vi "Get Controls RegisterMap.vi"(8 "error in (no error)":errorcluster, 11 "Item Ref in":T3 format="%.0x") -> (0 "error out":errorcluster, 2 "Controls RegisterMap":T1[](array[typedef]) {"fgpa cd ref" format="%.0x"; "reserver ref" format="%.0x"}, 3 "Item Ref out":T3 format="%.0x")   [LabVIEW 2016]
uses:
  <vilib>/NI VeriStand/Custom Device API/Custom Device API.lvlib
  <vilib>/NI Veristand/Custom Device API/Get Item Property (Variant).vi
  SubVIs/Channel Type.ctl
  FPGA Addon System Explorer.lvlib
  <vilib>/NI Veristand/Custom Device API/Custom Device Item Ref.ctl
  SubVIs/fpga resource.ctl
  VeriStand-FPGA-Resource-Manager/Source/FPGA Resource Manager System Definition.lvlib
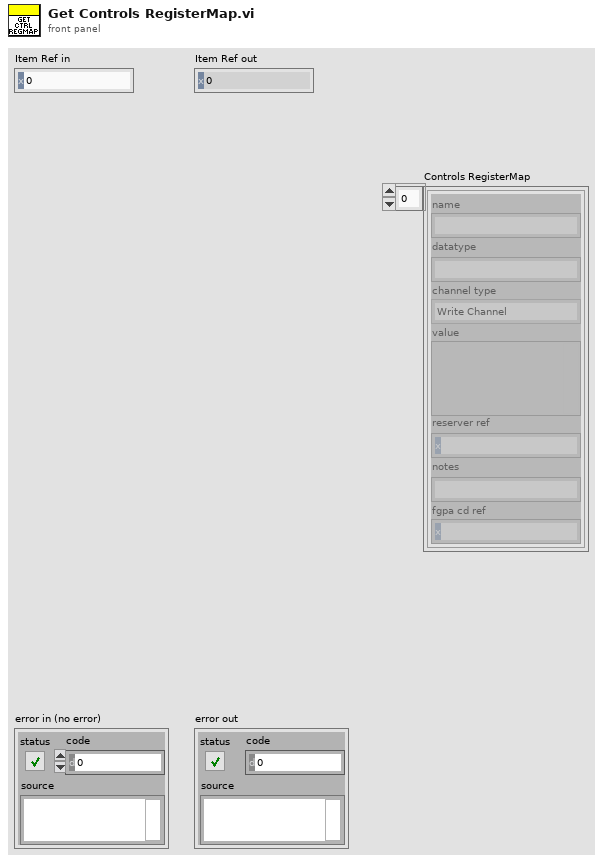
[diagram p1: front panel]
types:
  T1 = typedef "FPGA Addon System Explorer.lvlib/fpga resource.ctl" = cluster{"name":string, "datatype":string, "channel type":T2, "value":variant, "reserver ref":T3, "notes":string, "fgpa cd ref":T3}
  T2 = typedef "FPGA Addon System Explorer.lvlib/Channel Type.ctl" = enum16{"Write Channel", "Read Channel", "Write Waveform", "Read Waveform"}
  T3 = typedef "Custom Device API.lvlib/Custom Device Item Ref.ctl" = u64
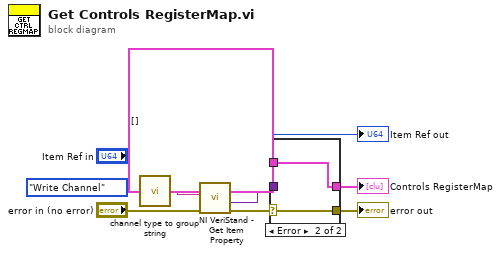
[diagram p0: block diagram]
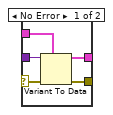
[diagram p2: hidden frame]
diagram:
  n1 = call "channel type to group string.vi"("channel type"=Channel_Type."Write Channel") -> ("FPGA.Controls"=w3:string)  [unwired: 10 in]
  n2 = call-poly <vilib>:"NI VeriStand - Get Item Property.vi"("error in (no error)"="error in (no error)", "Property Name"=w3, "Item Ref in"="Item Ref in") -> ("error out"=w6:errorcluster, "Value"=w7:variant, "Item Ref out"=→"Item Ref out":T3)  [unwired: 5 in, 1 out]
  n3 = case shown="Error" w6 {
    selector: w6 -> [w13 w16]
    tunnel: [w15 w17] -> w1
    tunnel: w7 -> [w14 _]
    tunnel: [w12 w16] -> w5
    tunnel: T1[] [] ("data") -> [w11 w17]
    frame No Error {
      n4 = Variant To Data(error in=w13, type=w11, Variant=w14) -> (data=w15:T1[], error out=w12:errorcluster)
    }
    frame Error {
    }
  }
  "error out" <- w5
  "Controls RegisterMap" <- w1
